vi "ms to samples.vi"(1 "ms":dbl) -> (0 "Samples":i32)   [LabVIEW 2014, in "Melody Extraction.lvlib"]
uses:
  Melody Extraction.lvlib
  dt_global.vi
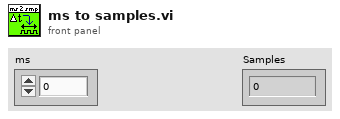
[diagram p1: front panel]
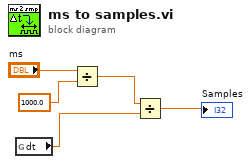
[diagram p0: block diagram]
diagram:
  n1 = global read "dt_global.vi" "dt"() -> (w2:dbl)
  n2 = Divide(x="ms", y=1000.0) -> (x/y=w3:dbl)
  n3 = Divide(x=w3, y=w2) -> (x/y=→"Samples":dbl)
